vi "Uim SFBK wrapper.vi"(8 "error in (no error)":errorcluster caption="错误输入（无错误）", 10 "dwCanNodeId":u32, 11 "dwDevIndex":u32) -> (0 "error out":errorcluster caption="错误输出", 2 "SFBK_INFO_OBJ":T1, 3 "function return":u32)   [LabVIEW 2016, in "UISimCanFunc_wrapper.lvlib"]
doc: "_declspec (dllexport) DWORD UimSFBK_wrapper(DWORD dwDevIndex, DWORD dwCanNodeId, P_SFBK_INFO_OBJ pSFBKInfo);"
uses:
  <userlib>/UISimCanFunc_wrapper/UISimCanFunc_wrapper.lvlib
  <userlib>/UISimCanFunc_wrapper/ctl/SFBK_INFO_OBJ.ctl
  <userlib>/UISimCanFunc_wrapper/UISimCanFunc_wrapper.dll
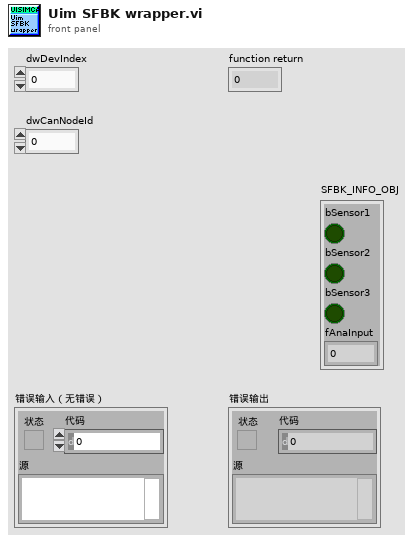
[diagram p1: front panel]
types:
  T1 = typedef "UISimCanFunc_wrapper.lvlib/SFBK_INFO_OBJ.ctl" = cluster{"bSensor1":bool, "bSensor2":bool, "bSensor3":bool, "fAnaInput":sgl}
  T2 = cluster{"bSensor1":i32, "bSensor2":i32, "bSensor3":i32, "fAnaInput":sgl}
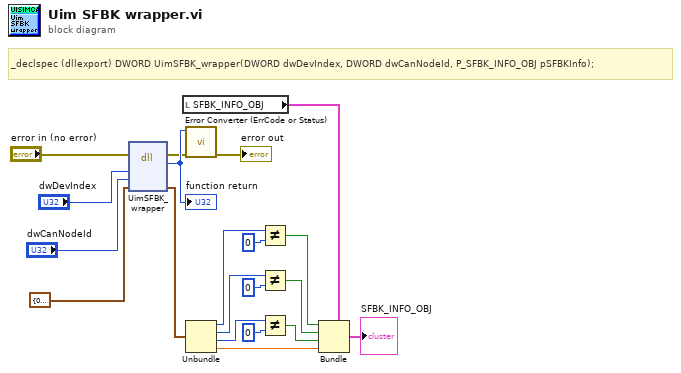
[diagram p0: block diagram]
diagram:
  # "_declspec (dllexport) DWORD UimSFBK_wrapper(DWORD dwDevIndex, DWORD dwCanNodeId, P_SFBK_INFO_OBJ pSFBKInfo);"
  n1 = dll-call lib="C:/Program Files (x86)/National Instruments/LabVIEW 2016/user.lib/UISimCanFunc_wrapper/UISimCanFunc_wrapper.*" fn="UimSFBK_wrapper"(error in="error in (no error)", "dwDevIndex"="dwDevIndex", "dwCanNodeId"="dwCanNodeId", "pSFBKInfo"=T2 {"bSensor1"=0, "bSensor2"=0, "bSensor3"=0, "fAnaInput"=0.0}) -> (error out=w15:errorcluster, w20:u32, "pSFBKInfo"=w12:T2)  [unwired: 4 in, 1 out]
  "function return" <- w20
  n2 = local read "SFBK_INFO_OBJ"() -> (w13:T1)
  n3 = call <userlib>:"Error Converter (ErrCode or Status).vi"("error in (no error)"=w15, "error code"=w20) -> ("error out"=→"error out":errorcluster)  [unwired: 9 in]
  n4 = Unbundle(w12) -> ("bSensor1"=w10:i32, "bSensor2"=w6:i32, "bSensor3"=w5:i32, "fAnaInput"=w2:sgl)
  n5 = Not Equal?(x=w10, y=0) -> (x != y?=w9:bool)
  n6 = Not Equal?(x=w6, y=0) -> (x != y?=w4:bool)
  n7 = Not Equal?(x=w5, y=0) -> (x != y?=w3:bool)
  n8 = Bundle(cluster=w13, "bSensor1"=w9, "bSensor2"=w4, "bSensor3"=w3, "fAnaInput"=w2) -> (→"SFBK_INFO_OBJ":T1)
